vi "Insert Main SubPanel.vi"(8 "error in (no error)":errorcluster, 9 "ActorQName":string, 10 "CalleeActorVI Ref":refnum<vi>, 11 "UI_Top in":refnum<class "UI_Top.lvclass">) -> (0 "error out":errorcluster, 3 "UI_Top out":refnum<class "UI_Top.lvclass">)   [LabVIEW 2021, in "UI_Top.lvclass"]
uses:
  UI_Top.lvclass
  UI_Top.lvclass/UI_Top.ctl
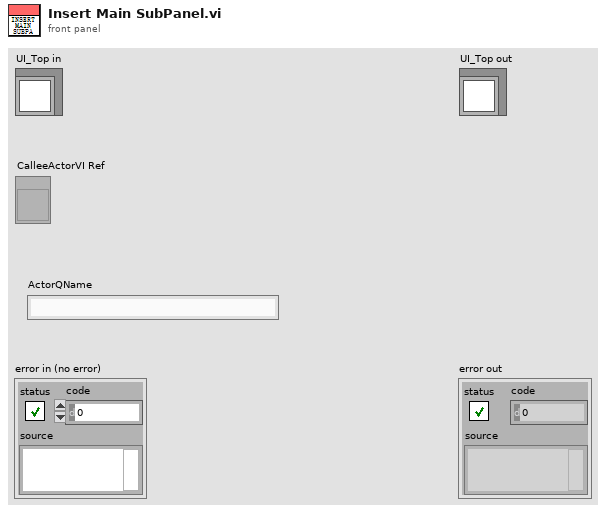
[diagram p1: front panel]
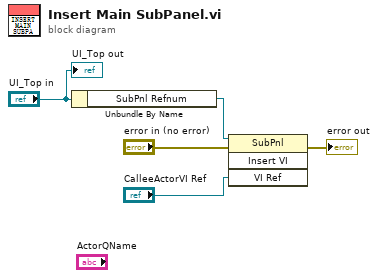
[diagram p0: block diagram]
diagram:
  n1 = Unbundle By Name("UI_Top in") -> ("SubPnl Refnum"=w4:refnum<vi>)
  n2 = invoke class="SubPnl" method="Insert VI"(reference=w4, error in="error in (no error)", "VI Ref"="CalleeActorVI Ref") -> (error out=→"error out":errorcluster)  [unwired: 1 in, 3 out]
  "UI_Top out" <- "UI_Top in"
